vi "Cluster Visualizer.vi"(10 "Array 2":T2(array[cluster]), 11 "Array in":cluster{"x":dbl, "y":dbl, dbl}[](array[cluster])) -> ()   [LabVIEW 2025]
uses:
  Framework/Robot Global Data.vi
panel:
  out "Front Point Cursor":T1
  in  "Robot Size (in)":cluster{"Width":dbl, "Length":dbl}
  out "Field":cluster{dbl[], dbl[]}[](graph)
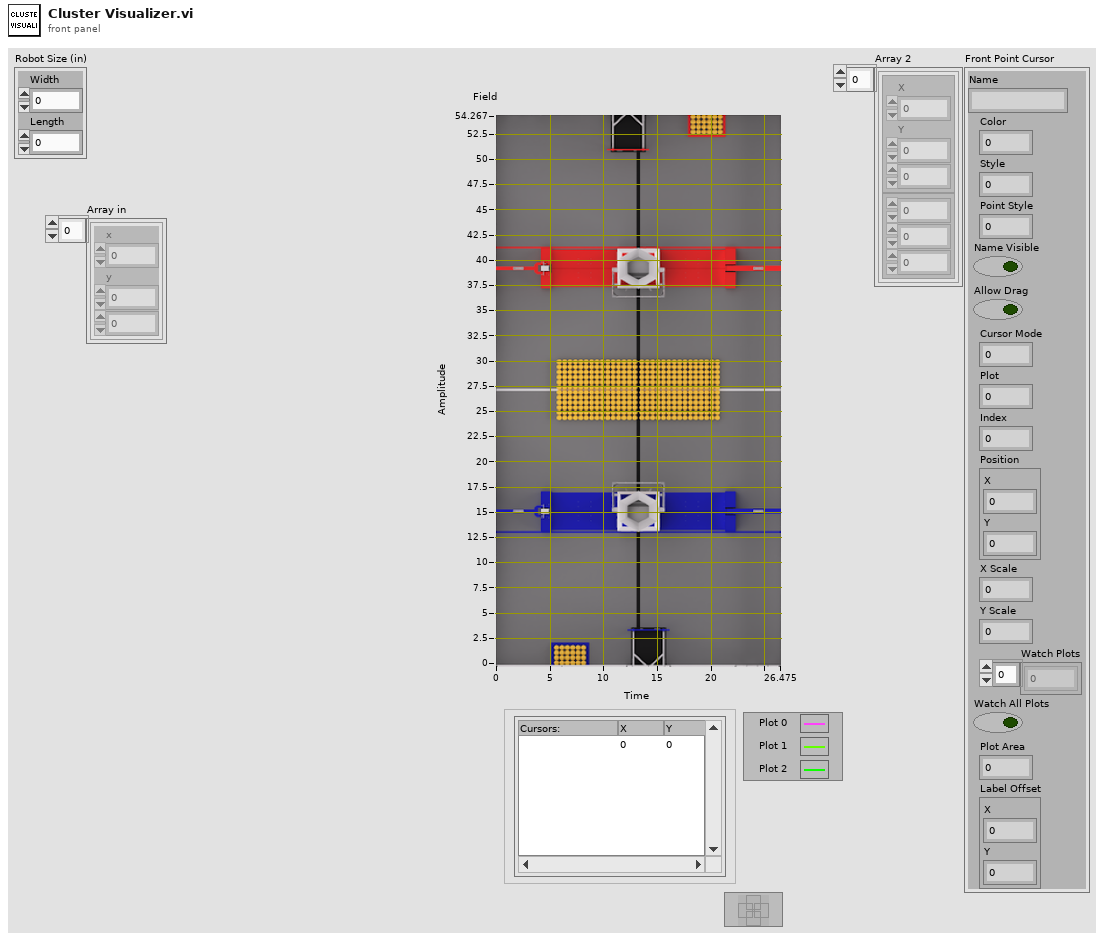
[diagram p1: front panel]
types:
  T1 = cluster{"Name":string, "Color":u32, "Style":i32, "Point Style":i32, "Name Visible":bool, "Allow Drag":bool, "Cursor Mode":u32, "Plot":i32, "Index":i32, "Position":cluster{"X":dbl, "Y":dbl}, "X Scale":u32, "Y Scale":u32, "Watch Plots":i32[], "Watch All Plots":bool, "Plot Area":i32, "Label Offset":cluster{"X":i32, "Y":i32}}
  T2 = cluster{cluster{"X":dbl, "Y":dbl, dbl}, cluster{dbl, dbl, dbl}}[]
  T3 = cluster{"Name":string, "Color":u32, "Style":i32, "Point Style":i32, "Name Visible":bool, "Allow Drag":bool, "Cursor Mode":u32, "Plot":i32, "Index":i32, "Position":cluster{"X":dbl, "Y":dbl}, "X Scale":u32, "Y Scale":u32, "Watch Plots":i32[], "Watch All Plots":bool, "Plot Area":i32, "Label Offset":cluster{"X":i32, "Y":i32}}[]
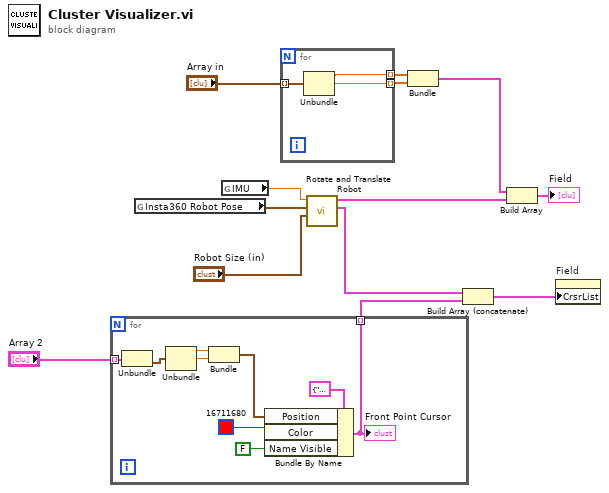
[diagram p0: block diagram]
diagram:
  n1 = for {
    tunnel: "Array 2" -> [w22] mode=indexing
    tunnel: [w14] -> w1 mode=indexing
    n2 = Unbundle(w22) -> (w21:cluster{dbl, dbl, dbl})  [unwired: 1 out]
    n3 = Unbundle(w21) -> (w20:dbl, w19:dbl)  [unwired: 1 out]
    n4 = Bundle(w20, w19) -> (w15:cluster{dbl, dbl})  [unwired: 1 in]
    n5 = Bundle By Name(cluster=T1 {"Name"="", "Color"=61192, "Style"=4, "Point Style"=6, "Name Visible"=TRUE, "Allow Drag"=TRUE, "Cursor Mode"=0, "Plot"=0, "Index"=0, "Position"={"X"=0.0, "Y"=0.0}, "X Scale"=0, "Y Scale"=0, "Watch Plots"=[], "Watch All Plots"=FALSE, "Plot Area"=0, "Label Offset"={"X"=1, "Y"=1}}, "Position"=w15, "Color"=u32 16711680, "Name Visible"=FALSE) -> (w14:T1)
    "Front Point Cursor" <- w14
  }
  n6 = global read "Robot Global Data.vi" "Insta360 Robot Pose"() -> (w4:cluster{"X":dbl, "Y":dbl})
  n7 = global read "Robot Global Data.vi" "IMU"() -> (w3:dbl)
  n8 = for {
    tunnel: "Array in" -> [w25] mode=indexing
    tunnel: [w24] -> w8 mode=indexing
    tunnel: [w23] -> w9 mode=indexing
    n9 = Unbundle(w25) -> ("x"=w24:dbl, "y"=w23:dbl)  [unwired: 1 out]
  }
  n10 = call "Rotate and Translate Robot.vi"("Robot Size (in)"="Robot Size (in)", "Robot Pose"=w4, "Theta"=w3) -> ("Front Point Cursor"=w12:T1, "output cluster"=w6:cluster{dbl[], dbl[]})  [unwired: 7 in]
  n11 = Bundle(w8, w9) -> (w7:cluster{dbl[], dbl[]})  [unwired: 1 in]
  n12 = Build Array (concatenate)(w12, w1) -> (w11:T3)
  n13 = Build Array(w7, w6) -> (→"Field":cluster{dbl[], dbl[]}[])
  n14 = property on="Field" class="XYGraph (strict)"("CrsrList"=w11) -> ()  [unwired: 2 in, 2 out]
